vi "Camera SelectionToggle Example.vi"() -> ()   [LabVIEW 2016]
uses:
  Global State Variables.vi
panel:
  out "Camera Selected":enum16{"Peg Camera", "Rope Camera"}(ring)
  in  "Button Ignore Timer":dbl
  in  "stop":bool
  in  "State Selector Methods":enum32{"using one button", "using two buttons"}(tab)
  in  "single buton selector":bool
  in  "right button\nselector":bool
  in  "left button \nselector":bool
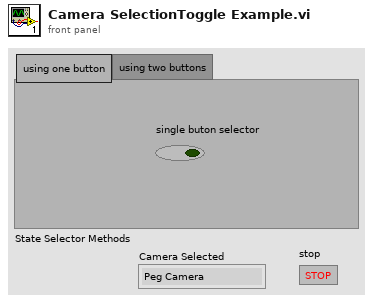
[diagram p1: front panel]
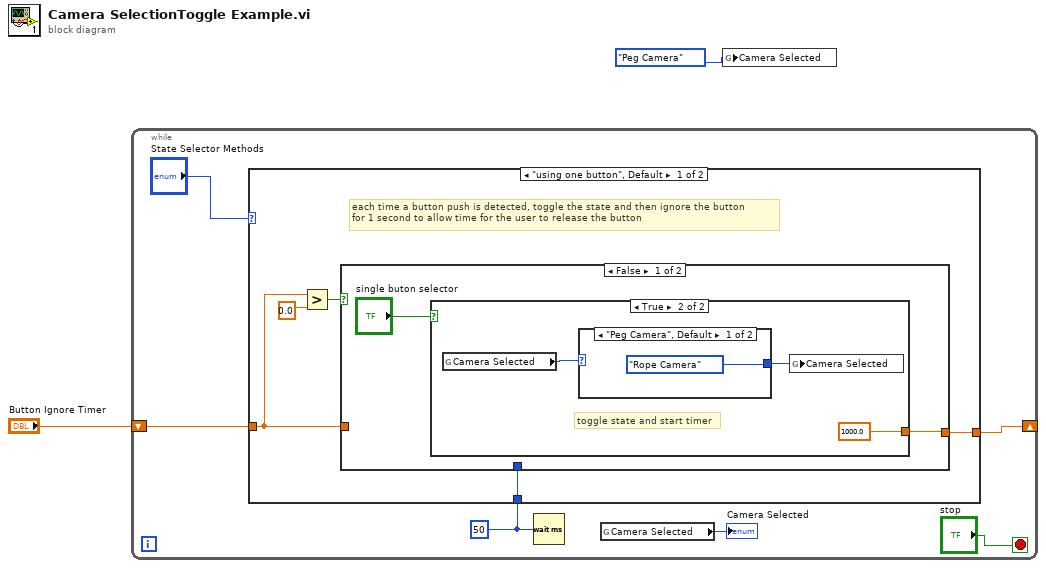
[diagram p0: block diagram]
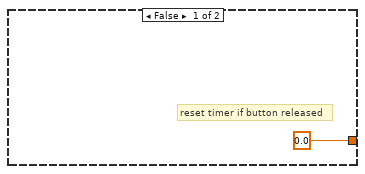
[diagram p2: hidden frame]
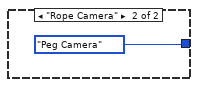
[diagram p3: hidden frame]
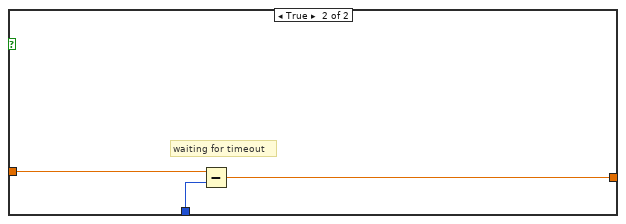
[diagram p4: hidden frame]
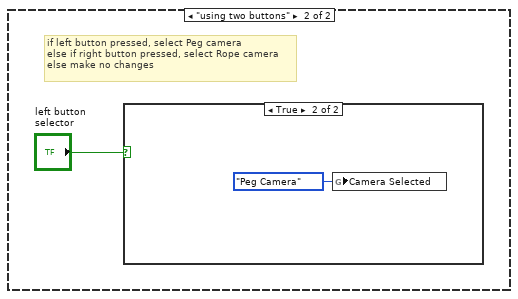
[diagram p5: hidden frame]
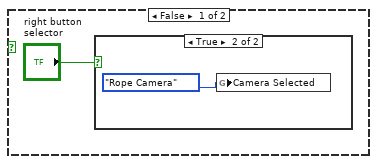
[diagram p6: hidden frame]
diagram:
  n1 = while {
    shift-right: [w4] -> _
    shift-left: "Button Ignore Timer" -> [w6]
    stop <- "stop" stop-if-true
    w5 = u32 50 ("milliseconds to wait")
    n2 = case shown="\"using one button\", Default" "State Selector Methods" {
      tunnel: w6 -> [w11 _]
      tunnel: w5 -> [w10 _]
      tunnel: [w9 _] -> w4
      frame "using one button", Default {
        # "each time a button push is detected, toggle the state and then ignore the button \nfor 1 second to allow time for the user to release the button"
        n3 = Greater?(x=w11, y=0.0) -> (0:w13:bool)
        n4 = case shown="False" w13 {
          tunnel: w11 -> [_ w23]
          tunnel: w10 -> [_ w24]
          tunnel: [w14 w22] -> w9
          frame False {
            n5 = case shown="True" "single buton selector" {
              tunnel: [0.0 ("Button Ignore Timer") 1000.0] -> w14
              frame False {
                # "reset timer if button released"
              }
              frame True {
                # "toggle state and start timer"
                n6 = global read "Global State Variables.vi" "Camera Selected"() -> (w19:enum16{"Peg Camera", "Rope Camera"})
                n7 = case shown="\"Peg Camera\", Default" w19 {
                  tunnel: [enum16{"Peg Camera", "Rope Camera"}."Rope Camera" ("Camera Selected") enum16{"Peg Camera", "Rope Camera"}."Peg Camera" ("Camera Selected")] -> w18
                  frame "Peg Camera", Default {
                  }
                  frame "Rope Camera" {
                  }
                }
                n8 = global write "Global State Variables.vi" "Camera Selected"(w18) -> ()
              }
            }
          }
          frame True {
            # "waiting for timeout"
            n9 = Subtract(x=w23, y=w24) -> (x-y=w22:dbl)
          }
        }
      }
      frame "using two buttons" {
        # "if left button pressed, select Peg camera\nelse if right button pressed, select Rope camera\nelse make no changes"
        n10 = case shown="True" "left button \nselector" {
          frame False {
            n11 = case shown="True" "right button\nselector" {
              frame False {
              }
              frame True {
                n12 = global write "Global State Variables.vi" "Camera Selected"(enum16{"Peg Camera", "Rope Camera"}."Rope Camera" ("Camera Selected")) -> ()
              }
            }
          }
          frame True {
            n13 = global write "Global State Variables.vi" "Camera Selected"(enum16{"Peg Camera", "Rope Camera"}."Peg Camera" ("Camera Selected")) -> ()
          }
        }
      }
    }
    n14 = Wait (ms)(milliseconds to wait=w5) -> ()  [unwired: 1 out]
    n15 = global read "Global State Variables.vi" "Camera Selected"() -> (→"Camera Selected":enum16{"Peg Camera", "Rope Camera"})
  }
  n16 = global write "Global State Variables.vi" "Camera Selected"(enum16{"Peg Camera", "Rope Camera"}."Peg Camera" ("Camera Selected")) -> ()
